vi "HandleMesurement.vi"(5 "Save?":bool, 7 "Measurement Directory":path, 8 "error in (no error)":errorcluster, 10 "Measure?":bool, 11 "Application Data":T1) -> (0 "error out":errorcluster)   [LabVIEW 2019]
uses:
  Typedefs/#cluster_ApplicationData.ctl
  Typedefs/Acquisition Thread/#cluster_AcqQueueData.ctl
  Typedefs/Acquisition Thread/#enum_AcquisitionTask.ctl
  Typedefs/Saving Thread/#cluster_SavingQueueData.ctl
  Typedefs/Saving Thread/#enum_SavingTask.ctl
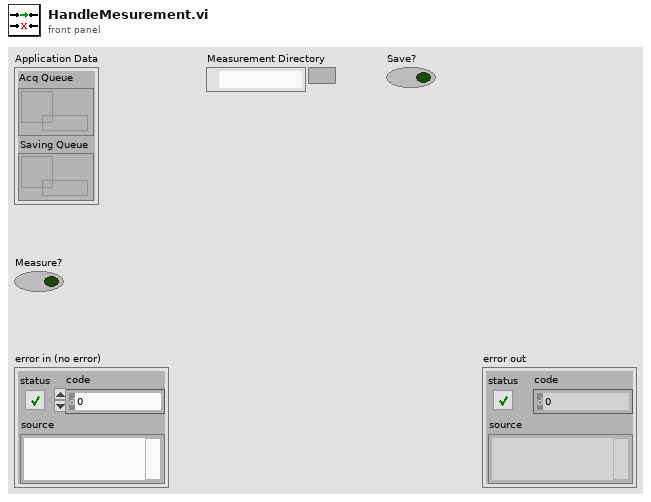
[diagram p1: front panel]
types:
  T1 = typedef "#cluster_ApplicationData.ctl" = cluster{"Acq Queue":refnum<queue>, "Saving Queue":refnum<queue>}
  T2 = typedef "#cluster_AcqQueueData.ctl" = cluster{"Task":T3, "Data":variant}
  T3 = typedef "#enum_AcquisitionTask.ctl" = enum16{"Init", "Start", "Finish", "Close"}
  T4 = typedef "#cluster_SavingQueueData.ctl" = cluster{"Task":T5, "Data":variant}
  T5 = typedef "#enum_SavingTask.ctl" = enum16{"Set directory", "Save", "Stop", "Close"}
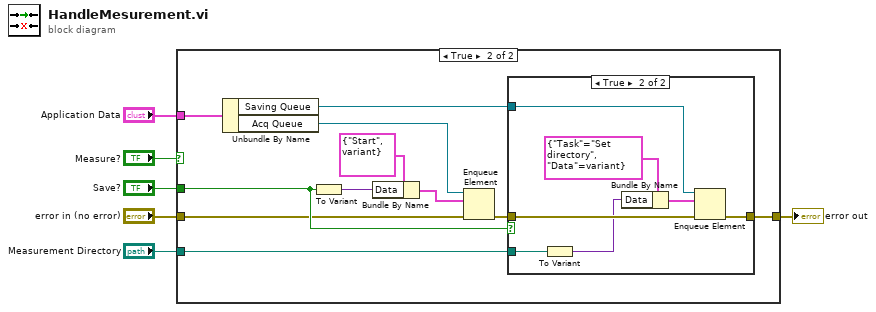
[diagram p0: block diagram]
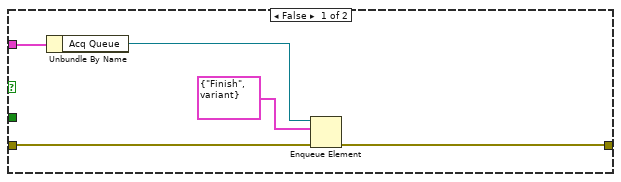
[diagram p2: hidden frame]
diagram:
  n1 = case shown="True" "Measure?" {
    tunnel: "error in (no error)" -> [w8 w12]
    tunnel: "Application Data" -> [w11 w22]
    tunnel: [w7 w15] -> w3
    tunnel: "Measurement Directory" -> [_ w14]
    tunnel: "Save?" -> [_ w13]
    frame False {
      n2 = Unbundle By Name(w11) -> ("Acq Queue"=w10:refnum<queue>)
      n3 = Enqueue Element(queue=w10, element=T2 {"Task"=enum."Finish", "Data"=variant}, error in (no error)=w8) -> (error out=w7:errorcluster)  [unwired: 1 in, 2 out]
    }
    frame True {
      n4 = Unbundle By Name(w22) -> ("Saving Queue"=w16:refnum<queue>, "Acq Queue"=w21:refnum<queue>)
      n5 = To Variant(anything=w13) -> (Variant=w19:variant)
      n6 = Bundle By Name(cluster=T2 {"Task"=enum."Start", "Data"=variant} ("element"), "Data"=w19) -> (w18:T2)
      n7 = Enqueue Element(queue=w21, element=w18, error in (no error)=w12) -> (error out=w17:errorcluster)  [unwired: 1 in, 2 out]
      n8 = case shown="True" w13 {
        tunnel: w17 -> [w23 w30]
        tunnel: w16 -> [_ w29]
        tunnel: w14 -> [_ w26]
        tunnel: [w23 w24] -> w15
        frame False {
        }
        frame True {
          n9 = To Variant(anything=w26) -> (Variant=w25:variant)
          n10 = Bundle By Name(cluster=T4 {"Task"=enum."Set directory", "Data"=variant} ("element"), "Data"=w25) -> (w27:T4)
          n11 = Enqueue Element(queue=w29, element=w27, error in (no error)=w30) -> (error out=w24:errorcluster)  [unwired: 1 in, 2 out]
        }
      }
    }
  }
  "error out" <- w3
